vi "CAN ISA Init.vi"(6 "Interrupt":T1(ring), 7 "BTR0BTR1(User)":i16 format="%.0x", 8 "Port":T2(ring)=enum."0x378", 9 "CAN Hw Type":enum16{"HW ISA (1)", "HW ISA SJA (9)"}(ring), 10 "CAN Msg Type":enum16{"11 Bit (0)", "29/11 Bit (1)"}(ring), 11 "BTR0BTR1":T3(ring)) -> (0 "IO_Port out":u32 format="%.0x", 1 "CANHwType out":i32, 2 "CANMsgType out":i32, 3 "BTR0BTR1 out":u16 format="%.0x", 4 "Interrupt out":u16, 5 "Error Number":u32)   [LabVIEW 2009]
doc: "Dieses VI initialisiert die CAN Hardware.\nAlle Eingabe sind durch ENUM Variablen\nrealisiert. Diese lassen sich in aufrufenden\nDiagrammen über die Funktion ´Creare Constant´\noder ´Create Control´ erzeugen.\n\nEingabe:\nBTR0BTR1: Baudratenregister. Einige Baudraten\n sind bereits vorgegeben. Eingene\n Einstellungen sind über den Eintrag\n ´User´ in der ENUM und die Belegung\n der Variablen ´ BTR0BTR1 (User)´ \n einstellbar.\nCAN Msg Type Einstellung ob 11 oder 29/11 bitt Identifier\nCAN Hw Type Auswahl der Hardware\nPort E/A Adresse\nInterrupt IRQ der Hardware\n\nAusgabe\nError Number Die Bedeutung steht im headerfile des\n Treibers. Leider steht in der Light Version\n des Treibers die in der Vollversion \n enthaltene Funktion zur ASusgabe des\n Fehlertextes nicht zur Verfügung.\nDie weiteren Ausgaben entsprechen den Eingaben. (Rückgabewerte der Treiber DLL)"
uses:
  PCAN_ISA.dll
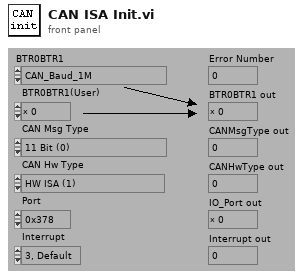
[diagram p1: front panel]
types:
  T1 = enum16{"3, Default", "4", "5", "7", "9", "10", "11", "12"}
  T2 = enum16{"0x100", "0x120", "0x140", "0x200", "0x220", "0x278", "0x2E8", "0x2F8", "0x300", "0x320", "0x340", "0x378", "0x38C", "0x3E8", "0x3F8", ""}
  T3 = enum16{"CAN_Baud_1M", "CAN_BAUD_500K", "CAN_BAUD_250K", "CAN_BAUD_125K", "CAN_BAUD_100K", "CAN_BAUD_50K", "CAN_BAUD_20K", "CAN_BAUD_10K", "CAN_BAUD_5K", "User"}
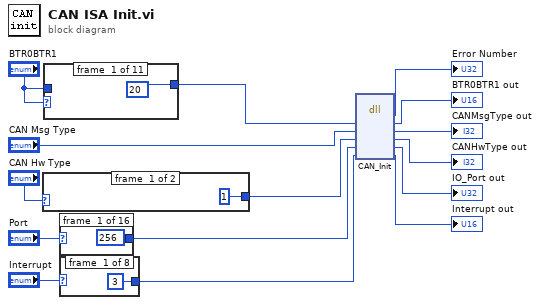
[diagram p0: block diagram]
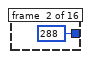
[diagram p2: hidden frame]
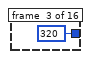
[diagram p3: hidden frame]
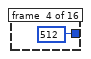
[diagram p4: hidden frame]
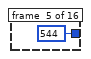
[diagram p5: hidden frame]
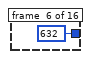
[diagram p6: hidden frame]
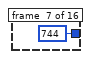
[diagram p7: hidden frame]
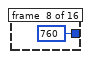
[diagram p8: hidden frame]
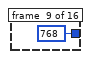
[diagram p9: hidden frame]
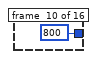
[diagram p10: hidden frame]
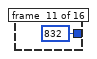
[diagram p11: hidden frame]
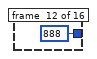
[diagram p12: hidden frame]
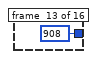
[diagram p13: hidden frame]
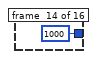
[diagram p14: hidden frame]
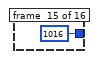
[diagram p15: hidden frame]
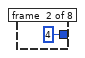
[diagram p17: hidden frame]
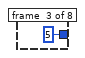
[diagram p18: hidden frame]
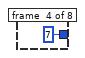
[diagram p19: hidden frame]
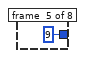
[diagram p20: hidden frame]
diagram:
  n1 = case shown="\"HW ISA SJA (9)\"" "CAN Hw Type" {
    tunnel: [1 9] -> w7
    frame #0 {
    }
    frame #1 {
    }
  }
  n2 = case shown="\"User\"" "BTR0BTR1" {
    tunnel: [i16 20 i16 28 i16 284 i16 796 i16 17199 i16 18223 i16 21295 i16 26415 i16 32639 "BTR0BTR1(User)" w28] -> w6
    tunnel: "BTR0BTR1" -> [_ _ _ _ _ _ _ _ _ _ w28]
    frame #0 {
    }
    frame #1 {
    }
    frame #2 {
    }
    frame #3 {
    }
    frame #4 {
    }
    frame #5 {
    }
    frame #6 {
    }
    frame #7 {
    }
    frame #8 {
    }
    frame #9 {
    }
    frame #10 {
    }
  }
  n3 = case shown="\"0x3F8\"" "Port" {
    selector: "Port" -> [_ _ _ _ _ _ _ _ _ _ _ _ _ _ _ w44]
    tunnel: [256 288 320 512 544 632 744 760 768 800 832 888 908 1000 1016 w44] -> w1
    frame #0 {
    }
    frame #1 {
    }
    frame #2 {
    }
    frame #3 {
    }
    frame #4 {
    }
    frame #5 {
    }
    frame #6 {
    }
    frame #7 {
    }
    frame #8 {
    }
    frame #9 {
    }
    frame #10 {
    }
    frame #11 {
    }
    frame #12 {
    }
    frame #13 {
    }
    frame #14 {
    }
    frame #15 {
    }
  }
  n4 = case shown="\"3, Default\", Default" "Interrupt" {
    tunnel: [3 4 5 7 9 10 11 12] -> w2
    frame #0 {
    }
    frame #1 {
    }
    frame #2 {
    }
    frame #3 {
    }
    frame #4 {
    }
    frame #5 {
    }
    frame #6 {
    }
    frame #7 {
    }
  }
  n5 = dll-call lib="C:/Documents and Settings/PQ/Desktop/LabView-Dateien/PCAN_ISA.dll" fn="CAN_Init"("BTR0BTR1"=w6, "CANMsgType"="CAN Msg Type", "CANHwType"=w7, "IO_Port"=w1, "Interrupt"=w2) -> (→"Error Number":u32, "BTR0BTR1"=→"BTR0BTR1 out":u16, "CANMsgType"=→"CANMsgType out":i32, "CANHwType"=→"CANHwType out":i32, "IO_Port"=→"IO_Port out":u32, "Interrupt"=→"Interrupt out":u16)  [unwired: 3 in, 2 out]
